vi "Remove ChildLink.vi"(8 "error in (no error)":errorcluster caption="错误输入（无错误）", 10 "ChildNode* in":refnum<data-value>, 11 "ParentLinkNode in":refnum<class "PanelLinkNode.lvclass"> caption="DNL_LabVIEW Object in") -> (0 "error out":errorcluster caption="错误输出", 3 "ParentLinkNode out":refnum<class "PanelLinkNode.lvclass"> caption="DNL_LabVIEW Object out")   [LabVIEW 2016, in "PanelLinkNode.lvclass"]
uses:
  PanelLinkNode.lvclass
  C:/Users/CL/Desktop/ZcDAQprj0811/ZcDAQprj/Modules/DAQ-Display/PanelSplitToolkit/PanelObject/PanelObject.lvclass
  PanelObject/PanelObject.lvclass
  PanelLinkNode.lvclass/PanelLinkNode.ctl
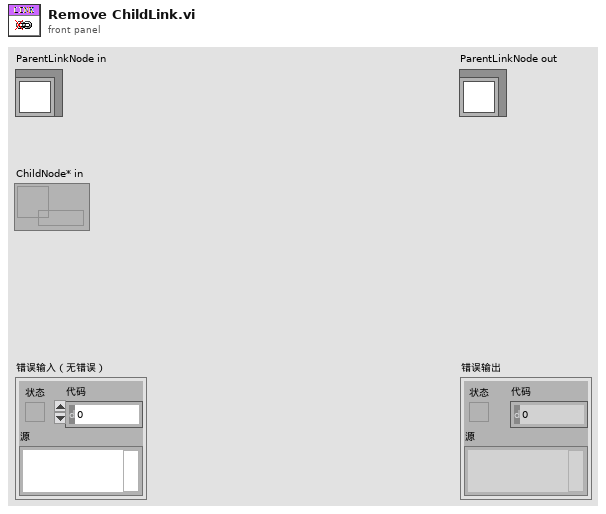
[diagram p1: front panel]
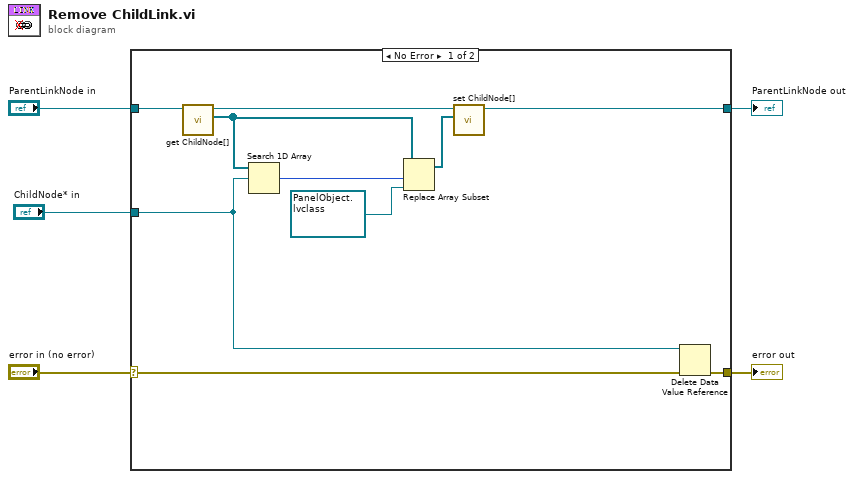
[diagram p0: block diagram]
diagram:
  n1 = case shown="No Error" "error in (no error)" {
    selector: "error in (no error)" -> [w7 w17]
    tunnel: [w15 w17] -> w4
    tunnel: [w9 w16] -> w2
    tunnel: "ParentLinkNode in" -> [w14 w16]
    tunnel: "ChildNode* in" -> [w8 _]
    frame No Error {
      n2 = call "get ChildNode[].vi"("PanelLinkNode输入"=w14) -> ("ChildNode*[]"=w13:refnum<data-value>[], "PanelLinkNode输出"=w10:refnum<class "PanelLinkNode.lvclass">)  [unwired: 8 in, 1 out]
      n3 = Search 1D Array(1D array=w13, element=w8) -> (index of element=w12:i32)  [unwired: 1 in]
      n4 = Replace Array Subset(array=w13, new element=refnum<data-value> refnum ("新元素/子数组"), index=w12) -> (w11:refnum<data-value>[])
      n5 = call "set ChildNode[].vi"("ChildNode*[]"=w11, "PanelLinkNode输入"=w10) -> ("PanelLinkNode输出"=w9:refnum<class "PanelLinkNode.lvclass">)  [unwired: 8 in, 1 out]
      n6 = Delete Data Value Reference(data value reference=w8, error in=w7) -> (error out=w15:errorcluster)  [unwired: 1 out]
    }
    frame Error {
    }
  }
  "error out" <- w4
  "ParentLinkNode out" <- w2
